vi "Send Last Clone Instance Notification.vi"(11 "Last Instance Notifier":refnum<notifier>) -> (0 "error out":errorcluster)   [LabVIEW 2024, in "Cloneable.lvlib" / "Clone Registration.lvlib"]
doc: "Fire the notifier to indicate that the last instance of a cloneable module is stopped.\n_____\nBased on DQMH Dev Tools: Project Template 7.1.0.1464."
uses:
  Clone Registration.lvlib
  Cloneable.lvlib
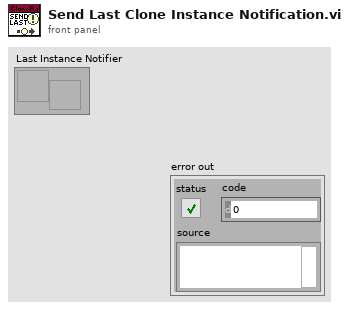
[diagram p1: front panel]
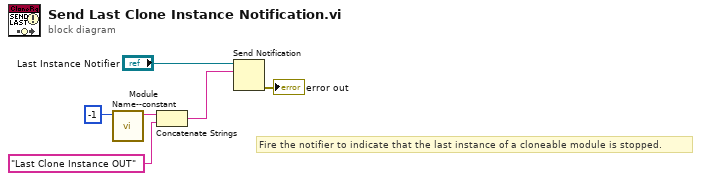
[diagram p0: block diagram]
diagram:
  # "Fire the notifier to indicate that the last instance of a cloneable module is stopped."
  n1 = call "Module Name--constant.vi"("Module ID"=-1) -> ("Module Name"=w2:string)  [unwired: 10 in]
  n2 = Concatenate Strings(w2, "Last Clone Instance OUT" ("string")) -> (w1:string)
  n3 = Send Notification(notification=w1, notifier="Last Instance Notifier") -> (error out=→"error out":errorcluster)  [unwired: 1 in, 1 out]
